vi "Rotate Raw.vi"(8 "error in":errorcluster, 9 "speed(deg/s)":dbl=2.0 min=0.0, 10 "position(deg)":dbl, 11 "Gantry in":refnum<class "Gantry.lvclass">) -> (0 "error out":errorcluster, 3 "Gantry out":refnum<class "Gantry.lvclass">)   [LabVIEW 2026, in "Gantry.lvclass"]
uses:
  Gantry.lvclass
  <instrlib>/Aerotech Automation1/Commands/Motion/typedefs/MoveAbsolute parameters.ctl
  FlexWorktable/FlexWorktable.lvclass
  <instrlib>/Aerotech Automation1/Aerotech Automation1.lvlib
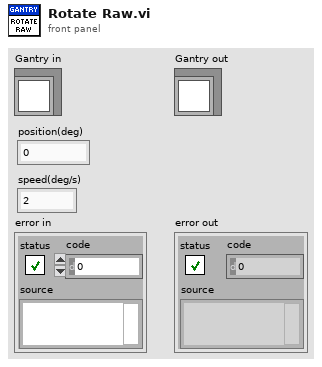
[diagram p1: front panel]
types:
  T1 = typedef "Aerotech Automation1.lvlib/MoveAbsolute parameters.ctl" = cluster{"speeds":dbl[], "positions":dbl[], "axes":string[]}
  T2 = typedef "Virtual Modes.ctl" = enum16{"Nonvirtual", "Virtual"}
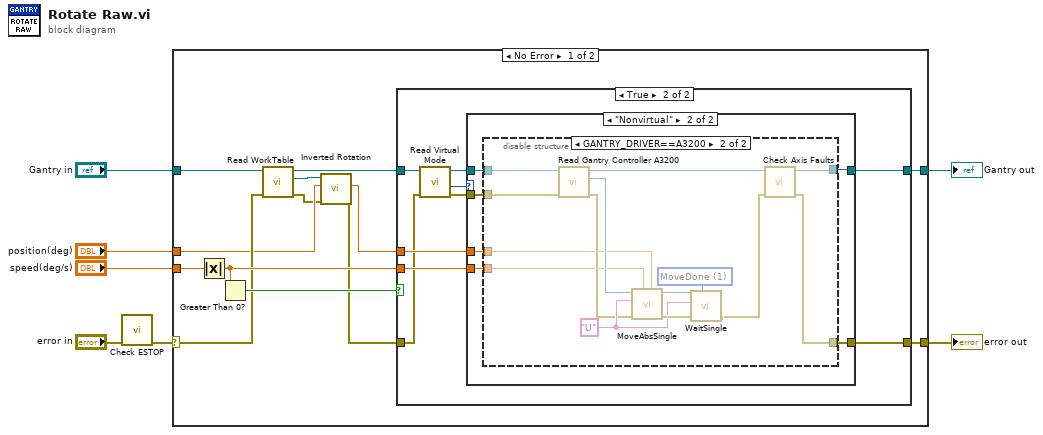
[diagram p0: block diagram]
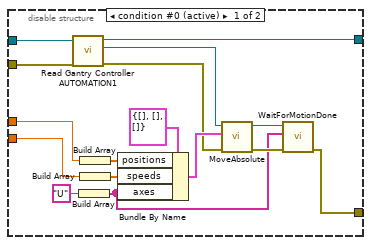
[diagram p4: hidden frame]
diagram:
  n1 = call "Check ESTOP.vi"("error in"="error in") -> ("error out"=w4:errorcluster)  [unwired: 10 in]
  n2 = case shown="No Error" w4 {
    selector: w4 -> [w14 w71]
    tunnel: [w20 w71] -> w7
    tunnel: [w17 w70] -> w6
    tunnel: "Gantry in" -> [w15 w70]
    tunnel: "position(deg)" -> [w11 _]
    tunnel: "speed(deg/s)" -> [w19 _]
    frame No Error {
      n3 = Absolute Value(x=w19) -> (abs(x)=w18:dbl)
      n4 = Greater Than 0?(x=w18) -> (x > 0?=w16:bool)
      n5 = call-dynamic "Read WorkTable.vi"("error in"=w14, "Gantry Class in"=w15) -> ("error out"=w9:errorcluster, "Worktable"=w12:refnum<class "FlexWorktable.lvclass">, "Gantry Class out"=w13:refnum<class "Gantry.lvclass">)  [unwired: 7 in]
      n6 = call "Inverted Rotation.vi"("error in (no error)"=w9, "Rotation in"=w11, "FlexWorktable in"=w12) -> ("error out"=w8:errorcluster, "Rotation out"=w10:dbl)  [unwired: 6 in, 1 out]
      n7 = case shown="True" w16 {
        tunnel: w13 -> [w22 w27]
        tunnel: w8 -> [w21 w25]
        tunnel: [w21 w31] -> w20
        tunnel: w10 -> [_ w30]
        tunnel: w18 -> [_ w29]
        tunnel: [w22 w28] -> w17
        frame False {
        }
        frame True {
          n8 = call-dynamic "Read Virtual Mode.vi"("error in (no error)"=w25, "Gantry in"=w27) -> ("error out"=w24:errorcluster, "Virtual Mode"=w23:T2, "Gantry out"=w26:refnum<class "Gantry.lvclass">)  [unwired: 6 in, 1 out]
          n9 = case shown="\"Nonvirtual\"" w23 {
            tunnel: w24 -> [w32 w38]
            tunnel: [w32 w35] -> w31
            tunnel: w30 -> [_ w37]
            tunnel: w29 -> [_ w36]
            tunnel: [w33 w34] -> w28
            tunnel: w26 -> [w33 w39]
            frame "Virtual" {
            }
            frame "Nonvirtual" {
              n10 = disable-structure shown="GANTRY_DRIVER==A3200" {
                disable-tunnel: w39 -> [w55 w58]
                disable-tunnel: w38 -> [w54 w59]
                disable-tunnel: w37 -> [w50 w61]
                disable-tunnel: w36 -> [w49 w60]
                disable-tunnel: [w41 w56] -> w35
                disable-tunnel: [w40 w57] -> w34
                frame condition #0 (active) {
                  n11 = call "Read Gantry Controller AUTOMATION1.vi"("error in (no error)"=w54, "Gantry in"=w55) -> ("error out"=w46:errorcluster, "Controller AUTOMATION1"=w45:refnum<k24>, "Gantry out"=w40:refnum<class "Gantry.lvclass">)  [unwired: 7 in]
                  n12 = Build Array("U") -> (w42:string[])
                  n13 = Build Array(w50) -> (w51:dbl[])
                  n14 = Build Array(w49) -> (w52:dbl[])
                  n15 = Bundle By Name(cluster=T1 {"speeds"=[], "positions"=[], "axes"=[]} ("MoveAbsolute parameters"), "positions"=w51, "speeds"=w52, "axes"=w42) -> (w47:T1)
                  n16 = call <instrlib>:"MoveAbsolute.vi"("error in (no error)"=w46, "MoveAbsolute parameters"=w47, "Controller Refnum"=w45) -> ("error out"=w43:errorcluster, "Controller Refnum out"=w44:refnum<k24>)  [unwired: 7 in]
                  n17 = call <instrlib>:"WaitForMotionDone.vi"("error in (no error)"=w43, "axes"=w42, "Controller Refnum"=w44) -> ("error out"=w41:errorcluster)  [unwired: 7 in, 1 out]
                }
                frame condition #1 {
                  w68 = 1 items=["InPosition", "MoveDone"] ("wait option?")
                  w66 = "U" ("axis name")
                  n18 = call "Read Gantry Controller A3200.vi"("error in (no error)"=w59, "Gantry in"=w58) -> ("error out"=w63:errorcluster, "A3200 controller out"=w62:refnum<k24>, "Gantry out"=w64:refnum<class "Gantry.lvclass">)  [unwired: 7 in]
                  n19 = call "MoveAbsSingle.vi"("position"=w61, "speed"=w60, "error in (no error)"=w63, "axis name"=w66, "controller in"=w62) -> ("error out"=w67:errorcluster, "controller out"=w69:refnum<k24>)  [unwired: 5 in]
                  n20 = call "WaitSingle.vi"("wait option?"=w68, "error in (no error)"=w67, "axis name"=w66, "controller in"=w69) -> ("error out"=w65:errorcluster)  [unwired: 5 in, 2 out]
                  n21 = call "Check Axis Faults.vi"("error in (no error)"=w65, "Gantry in"=w64) -> ("error out"=w56:errorcluster, "Gantry out"=w57:refnum<class "Gantry.lvclass">)  [unwired: 8 in]
                }
              }
            }
          }
        }
      }
    }
    frame Error {
    }
  }
  "error out" <- w7
  "Gantry out" <- w6
